vi "Frequency of the Nitrogen Probe (Set).vi"(6 "ISOBUS address":T4=-1 caption="ISOBUS address (-1)", 8 "error in":errorcluster, 9 "Unit":T1, 10 "Frequency Configuration":T5, 11 "Mercury Reference In":T6) -> (0 "error out":errorcluster, 2 "Response":T2, 3 "Mercury Reference Out":T6, 4 "Valid?":T3)   [LabVIEW 2013, in "Mercury iXX.lvlib" / "Level Meter.lvlib"]
doc: "Set the configuration for the Frequency of the nitrogen probe at both 0% and 100%."
uses:
  Level Meter.lvlib
  Private/Controls/Command Verbs.ctl
  Mercury iXX.lvlib
  Controls/Is Valid LED.ctl
  Controls/Comms Transport Layer.ctl
  Private/Controls/Query Dynamic Reference.ctl
  Controls/Mercury Reference.ctl
  Controls/ISOBus Address.ctl
  Controls/Response String.ctl
  Controls/Frequency Configuration.ctl
  Controls/Unit String.ctl
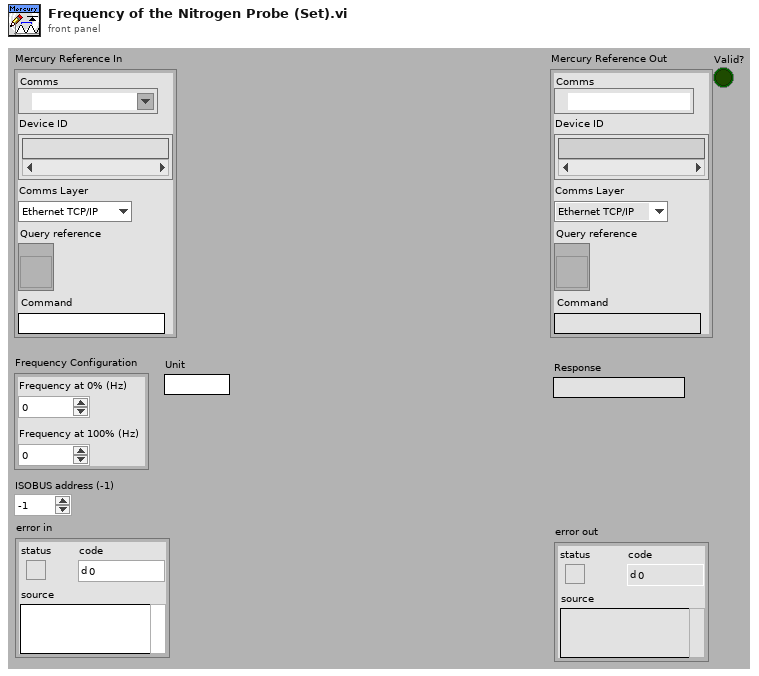
[diagram p1: front panel]
types:
  T1 = typedef "Mercury iXX.lvlib/Unit String.ctl" = string
  T2 = typedef "Mercury iXX.lvlib/Response String.ctl" = string
  T3 = typedef "Mercury iXX.lvlib/Is Valid LED.ctl" = bool
  T4 = typedef "Mercury iXX.lvlib/ISOBus Address.ctl" = i32
  T5 = typedef "Mercury iXX.lvlib/Level Meter.lvlib/Frequency Configuration.ctl" = cluster{"Freq 0%":dbl, "Freq 100%":dbl}
  T6 = typedef "Mercury iXX.lvlib/Mercury Reference.ctl" = cluster{"Comms":refnum<visa-resource-name>, "Device ID":string[], "Comms Layer":T7, "Command":string, "Query reference":T8}
  T7 = typedef "Mercury iXX.lvlib/Comms Transport Layer.ctl" = enum16{"Ethernet TCP/IP", "USB", "ISOBus - RS-232", "GPIB"}
  T8 = typedef "Mercury iXX.lvlib/Query Dynamic Reference.ctl" = refnum<vi>
  T9 = typedef "Mercury iXX.lvlib/Command Verbs.ctl" = string
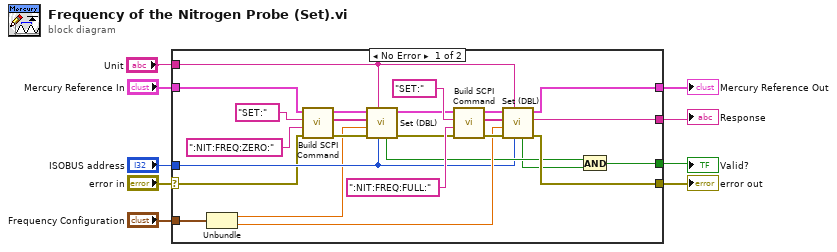
[diagram p0: block diagram]
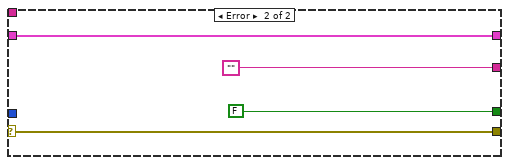
[diagram p2: hidden frame]
diagram:
  n1 = case shown="No Error" "error in" {
    selector: "error in" -> [w12 w38]
    tunnel: "Frequency Configuration" -> [w34 _]
    tunnel: "Mercury Reference In" -> [w28 w37]
    tunnel: [w19 w37] -> w5
    tunnel: [w18 w38] -> w2
    tunnel: "ISOBUS address" -> [w15 _]
    tunnel: [w14 T3 FALSE ("Valid?")] -> w3
    tunnel: [w13 ""] -> w4
    tunnel: "Unit" -> [w10 _]
    frame No Error {
      n2 = Unbundle(w34) -> ("Freq 0%"=w11:dbl, "Freq 100%"=w20:dbl)
      n3 = call "Build SCPI Command.vi"("error in"=w12, "Noun(s)"=":NIT:FREQ:ZERO:" ("Command"), "Verb"=T9 "SET:", "Mercury Reference In"=w28) -> ("error out"=w31:errorcluster, "SCPI Message(s)"=w29:string[], "Mercury Reference Out"=w30:T6)  [unwired: 5 out]
      n4 = call "Set (DBL).vi"("ISOBUS address"=w15, "Unit"=w10, "error in"=w31, "Command Value (Dbl)"=w11, "SCPI Message(s)"=w29, "Mercury Reference In"=w30) -> ("error out"=w22:errorcluster, "Mercury Reference Out"=w21:T6, "Valid?"=w17:T3)  [unwired: 3 out]
      n5 = call "Build SCPI Command.vi"("error in"=w22, "Noun(s)"=":NIT:FREQ:FULL:" ("Command"), "Verb"=T9 "SET:", "Mercury Reference In"=w21) -> ("error out"=w25:errorcluster, "SCPI Message(s)"=w23:string[], "Mercury Reference Out"=w24:T6)  [unwired: 5 out]
      n6 = call "Set (DBL).vi"("ISOBUS address"=w15, "Unit"=w10, "error in"=w25, "Command Value (Dbl)"=w20, "SCPI Message(s)"=w23, "Mercury Reference In"=w24) -> ("error out"=w18:errorcluster, "Response"=w13:T2, "Mercury Reference Out"=w19:T6, "Valid?"=w16:T3)  [unwired: 2 out]
      n7 = And(x=w17, y=w16) -> (x .and. y?=w14:T3)
    }
    frame Error {
    }
  }
  "Mercury Reference Out" <- w5
  "Valid?" <- w3
  "error out" <- w2
  "Response" <- w4
